vi "Enable TSTRB.vi"(10 "m_axis_tstrb":refnum<k21>, 11 "niInstr AXI4-Stream Reader FXP64x1 v1 FPGA in":refnum<class "niInstr AXI4-Stream Reader FXP64x1 v1 FPGA.lvclass">) -> (3 "niInstr AXI4-Stream Reader FXP64x1 v1 FPGA out":refnum<class "niInstr AXI4-Stream Reader FXP64x1 v1 FPGA.lvclass">)   [LabVIEW 2015, in "niInstr AXI4-Stream Reader FXP64x1 v1 FPGA.lvclass"]
doc: "Controls whether or not to generate TSTRB as part of the FPGA bitstream.\n\n<B>Input Parameters</B>\n\n<B>m_axis_tstrb</B> is the resource to use as TSTRB.\n\n<B>niInstr AXI4-Stream Reader FXP64x1 v1 FPGA in</B> takes in a reference to the AXI4-Stream Reader from the previous VI.\n\n<B>Output Parameters</B>\n\n<B>niInstr AXI4-Stream Reader FXP64x1 v1 FPGA out</B> passes a reference to the AXI4-Stream Reader to the next VI."
uses:
  <instrlib>/_niInstr/CLIP Adapters/v1/FPGA/AXI4-Stream/Reader FXP64x1/niInstr AXI4-Stream Reader FXP64x1 v1 FPGA.lvclass
  <instrlib>/_niInstr/CLIP Adapters/v1/FPGA/AXI4-Stream/Reader FXP64x1/niInstr AXI4-Stream Reader FXP64x1 v1 FPGA.lvclass/niInstr AXI4-Stream Reader FXP64x1 v1 FPGA.ctl
  <instrlib>/_niInstr/CLIP Adapters/v1/FPGA/AXI4-Stream/Reader/niInstr AXI4-Stream Reader v1 FPGA.lvclass
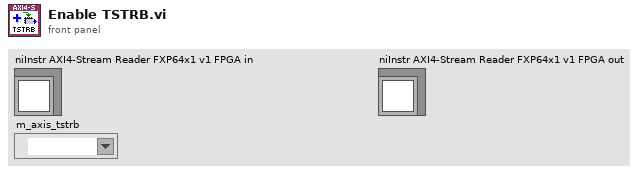
[diagram p1: front panel]
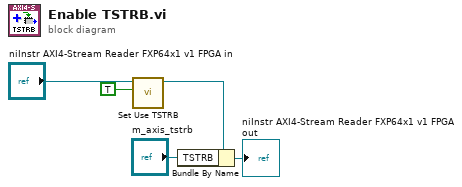
[diagram p0: block diagram]
diagram:
  n1 = call <instrlib>:"Set Use TSTRB.vi"("value"=TRUE ("Value"), "niInstr AXI4-Stream Reader v1 FPGA in"="niInstr AXI4-Stream Reader FXP64x1 v1 FPGA in") -> ("niInstr AXI4-Stream Reader v1 FPGA out"=w2:refnum<class "niInstr AXI4-Stream Reader FXP64x1 v1 FPGA.lvclass">)  [unwired: 9 in]
  n2 = Bundle By Name(cluster=w2, "TSTRB"="m_axis_tstrb") -> (→"niInstr AXI4-Stream Reader FXP64x1 v1 FPGA out":refnum<class "niInstr AXI4-Stream Reader FXP64x1 v1 FPGA.lvclass">)
